vi "Main v0.95.vi"() -> ()   [LabVIEW 2017]
doc: "v0.85:\n- Counts for rejects and total\n\nv0.5:\n\n- Added Reject to Manual Mode\n- Send reject pallet cluster during manual mode\n- Run continuous manual happens only when no error has occured"
uses:
  Controls/Main Tabs v0.1.ctl
  Controls/Auto.ctl
  RT/Controls/Auto Delays.ctl
  RT/Controls/Auto Times.ctl
  Controls/UI Data.ctl
  support/Controls/Auto Stats.ctl
  support/Message Queue/Enqueue Message (Single).vi
  GV/Maintenance GV.vi
  <vilib>/Utility/error.llb/Error Cluster From Error Code.vi
  <vilib>/ErrorRing/Error Ring.xnode
  support/Message Queue/Message Queue.lvlib
  support/User Event - Stop/User Event - Stop.lvlib
panel:
  in  "Reject Pallets":T1
  out "Date-Time":string caption="Dip-Tube Assembly Automation (HMI) v0.9"
  out "Main Tab":T2
  in  "Autocycle":T3
  in  "Manual":bool
  in  "Parameters":bool
  in  "Maintenance":bool
  in  "BF Para":cluster{"Delay 1":u32, "Delay 2":u32}={"Delay 1"=1000, "Delay 2"=1000}
  in  "Reject Para":cluster{"Delay":u32}={"Delay"=400}
  in  "Meas. Para":T4={"Delay"=500.0, "Mean Length"=188.9, "Tolerance"=1.0}
  in  "PF Para":cluster{"Delay":u32, "Timeout":u32}={"Delay"=1000, "Timeout"=1000}
  in  "Tube Feeder Para":T5={"Delay"=400, "Delay 2"=250, "Max Attempts"=250}
  in  "Cutting Para":T6={"Delay"=400, "Delay 2"=250, "Delay 3"=250}
  in  "Agitator Para":cluster{"Delay":u32, "Timeout":u32}={"Delay"=400, "Timeout"=250}
  in  "Insertion Para":cluster{"Delay 1":u32, "Delay 2":u32}={"Delay 1"=1000, "Delay 2"=1000}
  in  "Save Para":bool
  in  "Home Para":bool
  out "OEE":dbl format="%#.1f"
  out "QUA":dbl=100.0 min=0.0 max=100.0 step=0.1
  in  "Ideal Time":dbl=2.0 min=0.0 max=100.0 step=0.1
  in  "AVL":dbl=100.0 min=0.0 max=100.0 step=0.1
  out "Rejects 2":u32
  in  "Reset MCount":bool
  in  "Enable BF?":bool
  in  "Enable Agitate?":bool
  in  "Enable Reject?":bool
  in  "Toggle Motor":bool
  in  "Continuous?":bool
  in  "Enable Measure?":bool
  in  "Enable Index?":bool
  in  "Enable PF?":bool
  in  "Auto Para":T7={"Agitator Delays"=[400, 250], "TF Delays"=[700, 800, 2], "Insertion Delays"=[100, 500], "Cutting Delays"=[300, 300, 100], "PF Delays"=[250, 30000], "Measur. Delays"=[500.0, 188.9, 1.0], "Reject Delays"=[500], "BF Delays"=[1000, 1000]}
  in  "Enable Cutting?":bool
  in  "Enable Insertion?":bool
  in  "Run Manual":bool
  in  "Enable TF?":bool
  in  "Home Manual":bool
  out "Status 2":T9
  out "Measurements":T10 {"Height 1" format="%#.2f"; "Height 2" format="%#.2f"; "Height 3" format="%#.2f"; "Height 4" format="%#.2f"}
  out "Output Count":u32 caption="Output\nCount"
  out "PRF":dbl=100.0 min=0.0 max=100.0 step=0.1
  out "Statuses":string[][](table)
  in  "All IO":bool
  in  "Stats":bool
  in  "Home AC":bool
  out "Status":string
  out "Count":u32 format="%06.0f"
  out "Cycle Time":dbl format="%0.2f"
  out "Rejects":u32 format="%06.0f"
  out "Output Chart":T11(graph)
  out "Reject Count":u32
  out "Total Count":u32
  out "Total Time":dbl caption="Total Effective Cycle Time (s)" format="%#.3f"
  out "Time Chart":T12(graph)
  out "OEE Chart":cluster{"1":dbl, "2":dbl, "3":dbl, "4":dbl}(graph)
  out "Measurement Chart":cluster{"1":dbl, "2":dbl, "3":dbl, "4":dbl}(graph)
  out "Timestamp":string caption="Date & Timestamp"
  out "Latest Measure.":T13 caption="Latest Measurements" {"Length 1 (mm)" format="%#.2f"}
  out "Auto Times":T8
  in  "Back Stats":bool
  out "OEE 2":T14 caption="Latest Measurements" {"AVL" format="%#.1f"; "PRF" format="%#.1f"; "QUA" format="%#.1f"; "OEE" format="%#.1f"}
  out "IAS 4":dbl format="%#.3f"
  out "IAS 3":dbl format="%#.3f"
  out "IAS 2":dbl format="%#.3f"
  out "IAS 1":dbl format="%#.3f"
  out "DI 1":T15
  out "DI 2":T16
  out "DO 1":T17
  in  "Back IO":bool
  in  "Exit":bool
  # "Vision Harmony Dip-Tube Assembly Automation"
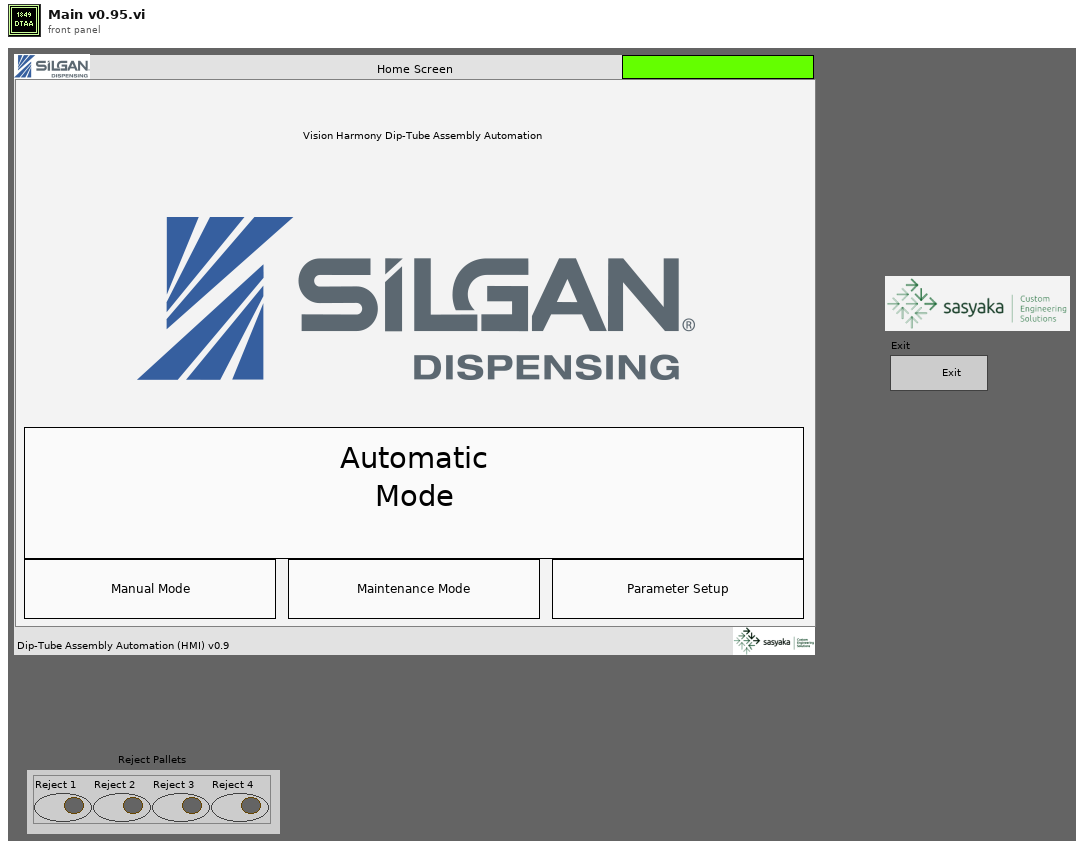
[diagram p1: front panel]
types:
  T1 = cluster{"Reject 1":bool, "Reject 2":bool, "Reject 3":bool, "Reject 4":bool}
  T2 = typedef "Main Tabs v0.1.ctl" = enum32{"Home Screen", "Parameter Setup", "Manual Mode", "Autocycle", "Autocycle Statistics", "Autocycle IOs"}
  T3 = typedef "Auto.ctl" = bool
  T4 = cluster{"Delay":dbl, "Mean Length":dbl, "Tolerance":dbl}
  T5 = cluster{"Delay":u32, "Delay 2":u32, "Max Attempts":u32}
  T6 = cluster{"Delay":u32, "Delay 2":u32, "Delay 3":u32}
  T7 = typedef "Auto Delays.ctl" = cluster{"Agitator Delays":u32[], "TF Delays":u32[], "Insertion Delays":u32[], "Cutting Delays":u32[], "PF Delays":u32[], "Measur. Delays":dbl[], "Reject Delays":u32[], "BF Delays":u32[]}
  T8 = typedef "Auto Times.ctl" = cluster{"Index Time":u32, "TF Time":u32, "Insertion Time":u32, "Cutting Time":u32, "PF Time":u32, "Meas. Time":u32, "Reject Time":u32}
  T9 = cluster{"Auto Times":T8, "error out":errorcluster}
  T10 = cluster{"Height 1":dbl, "Height 2":dbl, "Height 3":dbl, "Height 4":dbl}
  T11 = cluster{"OutputCount":u32, "Numeric Control":u32}
  T12 = cluster{"Index":dbl, "TF":dbl, "Insert":dbl, "Cutting":dbl, "PF":dbl, "Measure.":dbl, "Reject":dbl}
  T13 = cluster{"Length 1 (mm)":dbl, "Pallet 2 (mm)":dbl, "Pallet 3 (mm)":dbl, "Pallet 4 (mm)":dbl}
  T14 = cluster{"AVL":dbl, "PRF":dbl, "QUA":dbl, "OEE":dbl}
  T15 = cluster{"Machine_ON":bool, "E_stop ":bool, "SW_Pressure":bool, "SW_Start ":bool, "SW_Reset":bool, "SW_Stop":bool, "SW_Door":bool, "RS_Index_Rotary_CW":bool, "RS_Index_Rotary_CCW":bool, "RS_Index_Stopper _Rear":bool, "RS_Index_Output_Separator_Rear":bool, "PES_Index_Pallet_Sensor":bool, "PES_Index_Output_Part Sensor":bool, "ICS_BF_Low_Level_1":bool, "ICS_BF_Low_Level_2":bool, "ICS_BF_Pump_CNVR_Full_1":bool, "ICS_BF_Pump_CNVR_Full_2":bool, "ICS_BF_Pump_CNVR_Full_3":bool, "ICS_BF_Pump_CNVR_Full_4":bool, "PES_PC_Pump Presence_1":bool, "PES_PC_Pump Presence_2":bool, "PES_PC_Pump Presence_3":bool, "PES_PC_Pump Presence_4":bool, "RS_PC_Gating_Front":bool, "PES_Pump_Interference":bool, "PES_TF_Low_Level":bool, "PES_Tube Presence_1":bool, "PES_Tube Presence_2":bool, "PES_Tube Presence_3":bool, "PES_Tube Presence_4":bool, "DI1.30":bool, "DI1.31":bool}
  T16 = cluster{"RS_Agitatator_1_Rear ":bool, "RS_Agitatator_2_Rear ":bool, "RS_TF_Gating CYL_Rear":bool, "RS_Insertion_1_Rear":bool, "RS_Insertion_1_Front":bool, "RS_Insertion _2_Rear":bool, "RS_Insertion _2_Front":bool, "RS_Insertion _3_Rear":bool, "RS_Insertion _3_Front":bool, "RS_Insertion _4_Rear":bool, "RS_Insertion _4_Front":bool, "RS_Insertion_Clamp_Rear":bool, "RS_Cutting_Rear":bool, "RS_Cutting_Clamp _Rear":bool, "RS_Measurement_1_Rear":bool, "RS_Measurement_2_Rear":bool, "RS_Measurement_3_Rear":bool, "RS_Measurement_4_Rear":bool, "DI2.18":bool, "RS_Rejection_1_Rear":bool, "RS_Rejection_2_Rear":bool, "RS_Rejection_3_Rear":bool, "RS_Rejection_4_Rear":bool, "DI2.23":bool, "DI2.24":bool, "DI2.25":bool, "DI2.26":bool, "DI2.27":bool, "DI2.28":bool, "DI2.29":bool, "DI2.30":bool, "DI2.31":bool}
  T17 = cluster{"TL_Red":bool, "TL_Orange":bool, "TL_Green":bool, "TL_Buzzer":bool, "SOL_Index_Rotary_CW":bool, "SOL_Index_Rotary_CCW":bool, "SOL_Index_Stopper_Rear":bool, "SOL_OutputSeparator_Rear":bool, "Bowl  Feeder_ ON 1":bool, "Pump_CNVR_Motor _ON":bool, "SOL_PC_Gating_CYL_Rear":bool, "SOL_Tube_Feed_Agitatator":bool, "SOL_Tube_Feed_Gating_CYL":bool, "SOL_Insertion _CYL":bool, "SOL_Insertion_Clamp_CYL":bool, "SOL_Cutting_CYL":bool, "SOL_Cutting_Clamp_CYL":bool, "SOL_Insertion_Air_Nozzle":bool, "SOL_Measurement_CYL":bool, "DO1.19":bool, "SOL_Rejection CYL_1":bool, "SOL_Rejection CYL_2":bool, "SOL_Rejection CYL_3":bool, "SOL_Rejection CYL_4":bool, "Bowl  Feeder_ ON 2":bool, "SOL_BF_BlowerON":bool, "SOL_BF1_Track1":bool, "SOL_BF1_Track2":bool, "SOL_BF2_Track1":bool, "SOL_BF2_Track2":bool, "DO1.30":bool, "DO1.31":bool}
  T18 = typedef "UI Data.ctl" = cluster{"Main Tab":refnum<vi>}
  T19 = typedef "Message Queue.lvlib/All Message Queues.ctl" = cluster{"UI":refnum<queue>}
  T20 = enum8{"Enabled", "Disabled", "Disabled and Grayed Out"}
  T21 = cluster{"Array":string[][], "Machine Status":string}
  T22 = typedef "Auto Stats.ctl" = cluster{"Time":timestamp, "OEE":cluster{"AVL":dbl, "PRF":dbl, "QUA":dbl, "OEE":dbl}, "Auto Times":T8, "Counts out":cluster{"OutputCount":u32, "RejectCount":u32}, "Measurements":cluster{"1":dbl, "2":dbl, "3":dbl, "4":dbl}, "Outputs":cluster{"OutputCount":u32, "Numeric Control":u32}}
  T23 = cluster{"Auto Times":T8, "Results":cluster{"Measurements":cluster{"1":dbl, "2":dbl, "3":dbl, "4":dbl}, "Reject Pallets":cluster{"Reject 1":bool, "Reject 2":bool, "Reject 3":bool, "Reject 4":bool}}, "OutputCount":u32, "error out":errorcluster}
  T24 = cluster{"Agitator Delays[0]":u32, "Agitator Delays[1]":u32}
  T25 = cluster{"TF Delays[0]":u32, "TF Delays[1]":u32, "TF Delays[2]":u32}
  T26 = cluster{"Insertion Delays[0]":u32, "Insertion Delays[1]":u32}
  T27 = cluster{"Cutting Delays[0]":u32, "Cutting Delays[1]":u32, "Cutting Delays[2]":u32}
  T28 = cluster{"Measur. Delays[0]":dbl, "Measur. Delays[1]":dbl, "Measur. Delays[2]":dbl}
  T29 = typedef "All Inputs.ctl" = cluster{"DI 1":cluster{"Machine_ON":bool, "E_stop ":bool, "SW_Pressure":bool, "SW_Start ":bool, "SW_Reset":bool, "SW_Stop":bool, "SW_Door":bool, "RS_Index_Rotary_CW":bool, "RS_Index_Rotary_CCW":bool, "RS_Index_Stopper _Rear":bool, "RS_Index_Output_Separator_Rear":bool, "PES_Index_Pallet_Sensor":bool, "PES_Index_Output_Part Sensor":bool, "ICS_BF_Low_Level_1":bool, "ICS_BF_Low_Level_2":bool, "ICS_BF_Pump_CNVR_Full_1":bool, "ICS_BF_Pump_CNVR_Full_2":bool, "ICS_BF_Pump_CNVR_Full_3":bool, "ICS_BF_Pump_CNVR_Full_4":bool, "PES_PC_Pump Presence_1":bool, "PES_PC_Pump Presence_2":bool, "PES_PC_Pump Presence_3":bool, "PES_PC_Pump Presence_4":bool, "RS_PC_Gating_Front":bool, "PES_Pump_Interference":bool, "PES_TF_Low_Level":bool, "PES_Tube Presence_1":bool, "PES_Tube Presence_2":bool, "PES_Tube Presence_3":bool, "PES_Tube Presence_4":bool, "DI1.30":bool, "DI1.31":bool}, "DI 2":cluster{"RS_Agitatator_1_Rear ":bool, "RS_Agitatator_2_Rear ":bool, "RS_TF_Gating CYL_Rear":bool, "RS_Insertion_1_Rear":bool, "RS_Insertion_1_Front":bool, "RS_Insertion _2_Rear":bool, "RS_Insertion _2_Front":bool, "RS_Insertion _3_Rear":bool, "RS_Insertion _3_Front":bool, "RS_Insertion _4_Rear":bool, "RS_Insertion _4_Front":bool, "RS_Insertion_Clamp_Rear":bool, "RS_Cutting_Rear":bool, "RS_Cutting_Clamp _Rear":bool, "RS_Measurement_1_Rear":bool, "RS_Measurement_2_Rear":bool, "RS_Measurement_3_Rear":bool, "RS_Measurement_4_Rear":bool, "RS_Measure_Clamp_Rear":bool, "RS_Rejection_1_Rear":bool, "RS_Rejection_2_Rear":bool, "RS_Rejection_3_Rear":bool, "RS_Rejection_4_Rear":bool, "DI2.23":bool, "DI2.24":bool, "DI2.25":bool, "DI2.26":bool, "DI2.27":bool, "DI2.28":bool, "DI2.29":bool, "DI2.30":bool, "DI2.31":bool}, "IAS 1":dbl, "IAS 2":dbl, "IAS 3":dbl, "IAS 4":dbl, "DO 1":cluster{"TL_Red":bool, "TL_Orange":bool, "TL_Green":bool, "TL_Buzzer":bool, "SOL_Index_Rotary_CW":bool, "SOL_Index_CNVR_Rotary_CCW":bool, "SOL_Index_CNVR_Stopper_Rear":bool, "SOL_Index_CNVR_Output _Separator _Rear":bool, "Bowl  Feeder_ ON 1":bool, "Pump_CNVR_Motor _ON":bool, "SOL_PC_Gating_CYL_Rear":bool, "SOL_Tube_Feed_Agitatator":bool, "SOL_Tube_Feed_Gating_CYL":bool, "SOL_Insertion _CYL":bool, "SOL_Insertion_Clamp_CYL":bool, "SOL_Cutting_CYL":bool, "SOL_Cutting_Clamp_CYL":bool, "SOL_Insertion_Air_Nozzle":bool, "SOL_Measurement_CYL":bool, "DO1.19":bool, "SOL_Rejection CYL_1":bool, "SOL_Rejection CYL_2":bool, "SOL_Rejection CYL_3":bool, "SOL_Rejection CYL_4":bool, "Bowl  Feeder_ ON 2":bool, "SOL_BF_BlowerON":bool, "SOL_BF1_Track1":bool, "SOL_BF1_Track2":bool, "SOL_BF2_Track1":bool, "SOL_BF2_Track2":bool, "DO1.30":bool, "DO1.31":bool}}
  T30 = cluster{"RS_Agitatator_1_Rear ":bool, "RS_Agitatator_2_Rear ":bool, "RS_TF_Gating CYL_Rear":bool, "RS_Insertion_1_Rear":bool, "RS_Insertion_1_Front":bool, "RS_Insertion _2_Rear":bool, "RS_Insertion _2_Front":bool, "RS_Insertion _3_Rear":bool, "RS_Insertion _3_Front":bool, "RS_Insertion _4_Rear":bool, "RS_Insertion _4_Front":bool, "RS_Insertion_Clamp_Rear":bool, "RS_Cutting_Rear":bool, "RS_Cutting_Clamp _Rear":bool, "RS_Measurement_1_Rear":bool, "RS_Measurement_2_Rear":bool, "RS_Measurement_3_Rear":bool, "RS_Measurement_4_Rear":bool, "RS_Measure_Clamp_Rear":bool, "RS_Rejection_1_Rear":bool, "RS_Rejection_2_Rear":bool, "RS_Rejection_3_Rear":bool, "RS_Rejection_4_Rear":bool, "DI2.23":bool, "DI2.24":bool, "DI2.25":bool, "DI2.26":bool, "DI2.27":bool, "DI2.28":bool, "DI2.29":bool, "DI2.30":bool, "DI2.31":bool}
  T31 = cluster{"TL_Red":bool, "TL_Orange":bool, "TL_Green":bool, "TL_Buzzer":bool, "SOL_Index_Rotary_CW":bool, "SOL_Index_CNVR_Rotary_CCW":bool, "SOL_Index_CNVR_Stopper_Rear":bool, "SOL_Index_CNVR_Output _Separator _Rear":bool, "Bowl  Feeder_ ON 1":bool, "Pump_CNVR_Motor _ON":bool, "SOL_PC_Gating_CYL_Rear":bool, "SOL_Tube_Feed_Agitatator":bool, "SOL_Tube_Feed_Gating_CYL":bool, "SOL_Insertion _CYL":bool, "SOL_Insertion_Clamp_CYL":bool, "SOL_Cutting_CYL":bool, "SOL_Cutting_Clamp_CYL":bool, "SOL_Insertion_Air_Nozzle":bool, "SOL_Measurement_CYL":bool, "DO1.19":bool, "SOL_Rejection CYL_1":bool, "SOL_Rejection CYL_2":bool, "SOL_Rejection CYL_3":bool, "SOL_Rejection CYL_4":bool, "Bowl  Feeder_ ON 2":bool, "SOL_BF_BlowerON":bool, "SOL_BF1_Track1":bool, "SOL_BF1_Track2":bool, "SOL_BF2_Track1":bool, "SOL_BF2_Track2":bool, "DO1.30":bool, "DO1.31":bool}
  T32 = cluster{"Auto Para":T7, "Reject Pallets":cluster{"Reject 1":bool, "Reject 2":bool, "Reject 3":bool, "Reject 4":bool}}
  T33 = cluster{"Measurements":cluster{"1":dbl, "2":dbl, "3":dbl, "4":dbl}, "Reject Pallets":cluster{"Reject 1":bool, "Reject 2":bool, "Reject 3":bool, "Reject 4":bool}}
  T34 = cluster{"Reject Pallets":cluster{"Reject 1":bool, "Reject 2":bool, "Reject 3":bool, "Reject 4":bool}, "Measurements":cluster{"1":dbl, "2":dbl, "3":dbl, "4":dbl}}
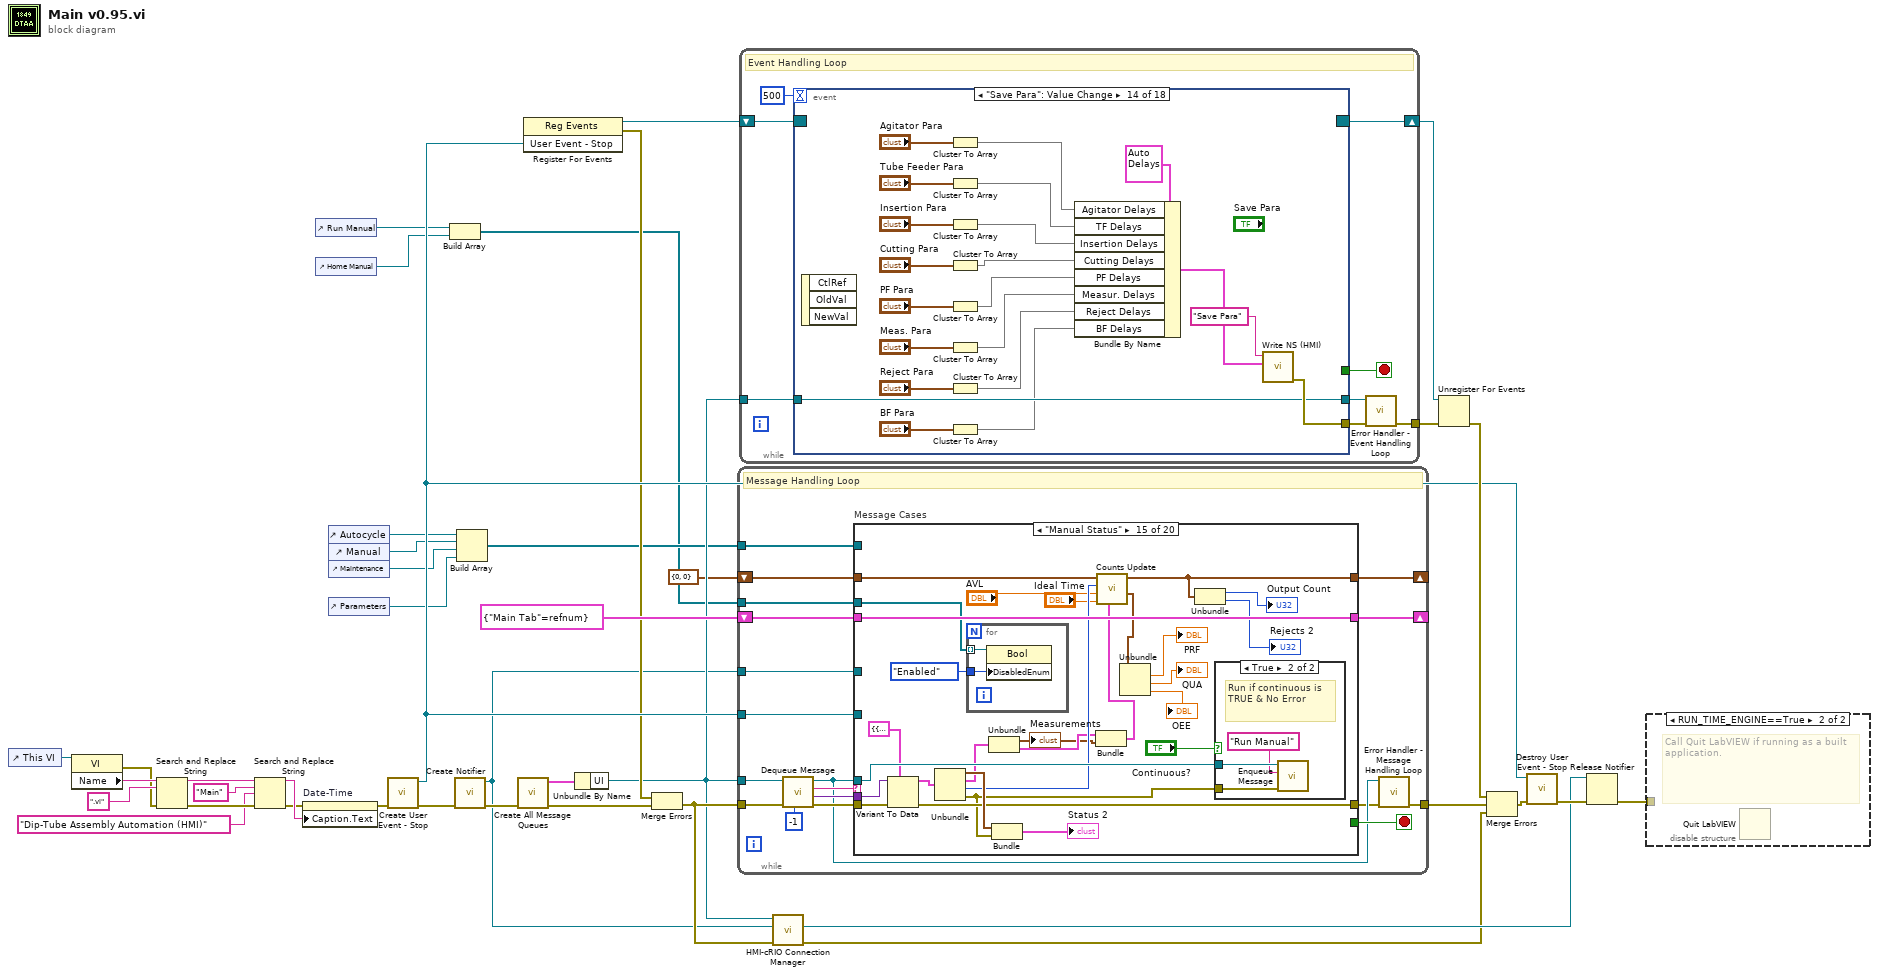
[diagram p0: block diagram]
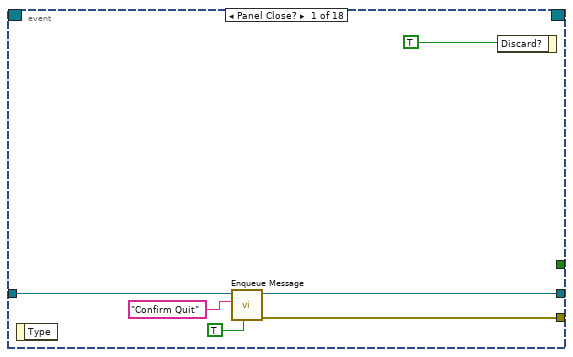
[diagram p2: hidden frame]
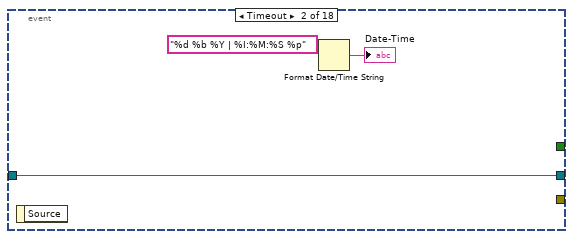
[diagram p3: hidden frame]
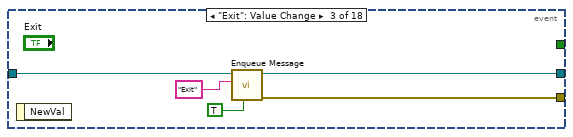
[diagram p4: hidden frame]
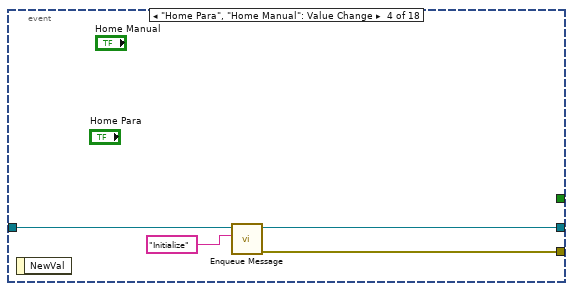
[diagram p5: hidden frame]
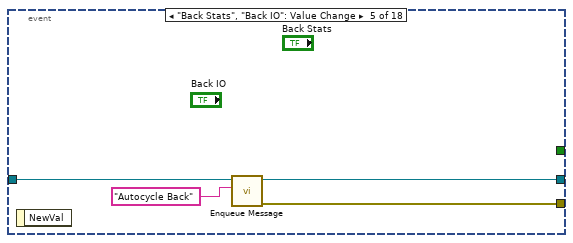
[diagram p6: hidden frame]
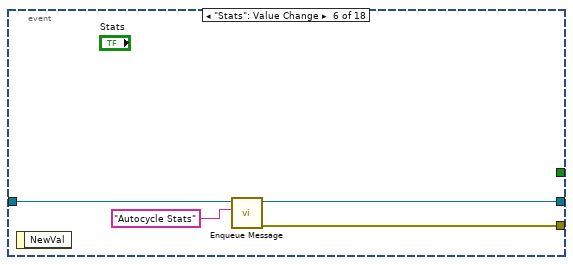
[diagram p7: hidden frame]
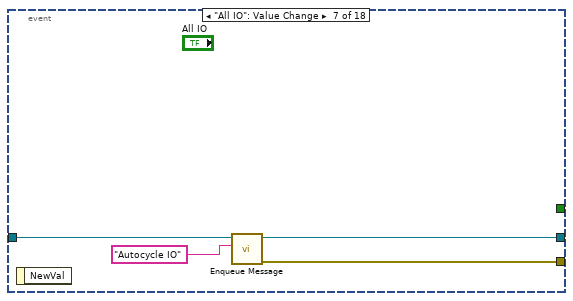
[diagram p8: hidden frame]
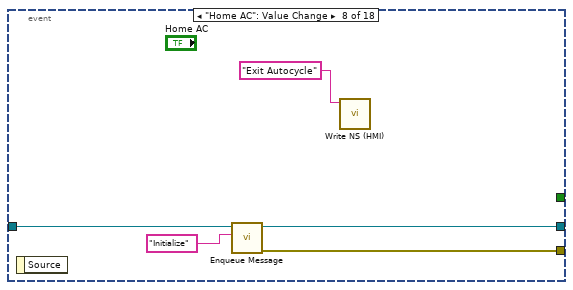
[diagram p9: hidden frame]
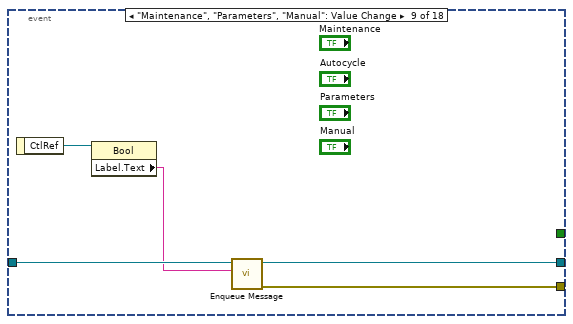
[diagram p10: hidden frame]
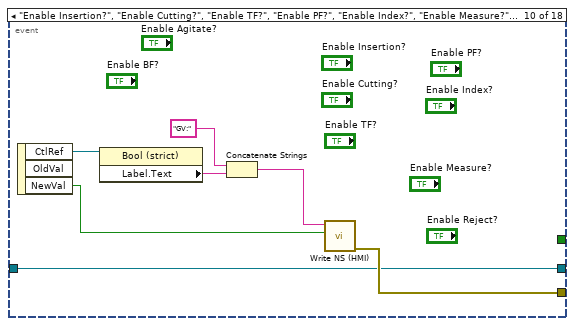
[diagram p11: hidden frame]
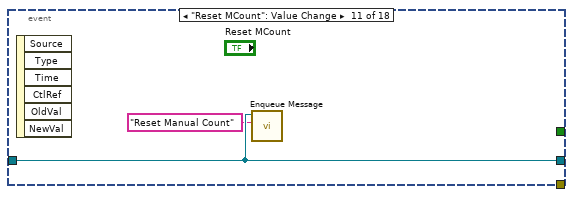
[diagram p12: hidden frame]
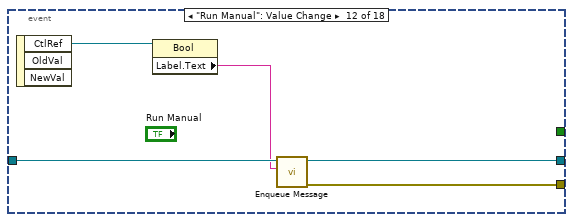
[diagram p13: hidden frame]
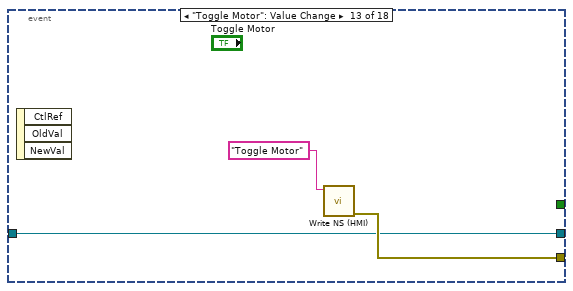
[diagram p14: hidden frame]
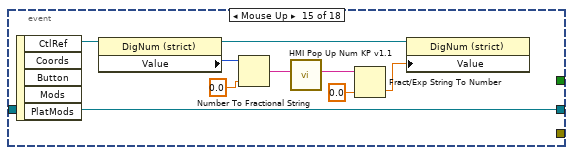
[diagram p15: hidden frame]
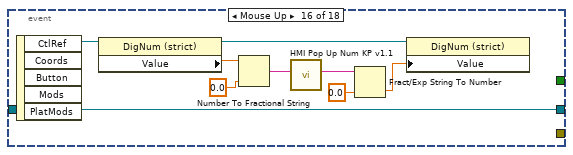
[diagram p16: hidden frame]
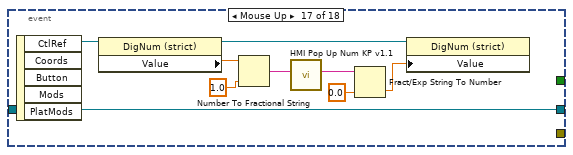
[diagram p17: hidden frame]
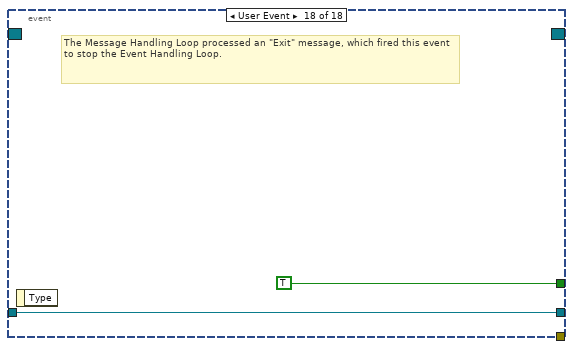
[diagram p18: hidden frame]
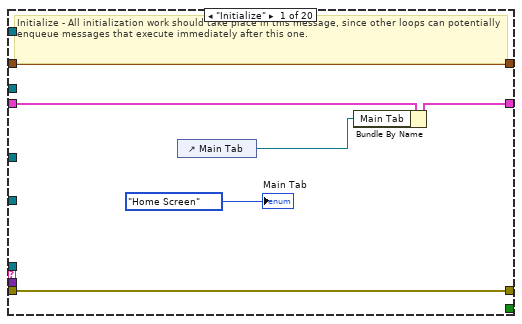
[diagram p19: hidden frame]
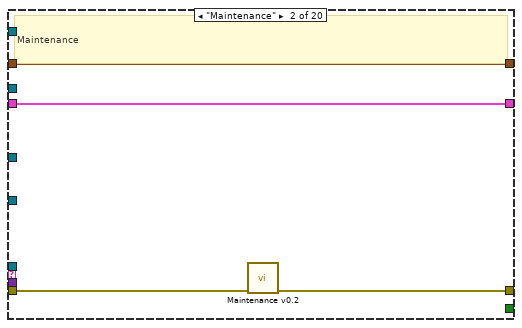
[diagram p20: hidden frame]
diagram:
  n1 = control-ref of="This VI"() -> (w9:refnum<vi>)
  n2 = property class="VI"(reference=w9) -> (error out=w8:errorcluster, "Name"=w15:string)  [unwired: 1 in, 1 out]
  n3 = Search and Replace String(input string=w15, search string=".vi", error in=w8) -> (result string=w13:string, error out=w12:errorcluster)  [unwired: 5 in, 2 out]
  n4 = Search and Replace String(input string=w13, search string="Main", replace string="Dip-Tube Assembly Automation (HMI)" ("replace string (\"\")"), error in=w12) -> (result string=w7:string, error out=w6:errorcluster)  [unwired: 4 in, 2 out]
  n5 = property on="Date-Time" class="Str"(error in=w6, "Caption.Text"=w7) -> (error out=w5:errorcluster)  [unwired: 1 in, 1 out]
  n6 = control-ref of="Run Manual"() -> (w4:refnum<vi>)
  n7 = control-ref of="Home Manual"() -> (w3:refnum<vi>)
  n8 = control-ref of="Autocycle"() -> (w20:refnum<vi>)
  n9 = control-ref of="Manual"() -> (w19:refnum<vi>)
  n10 = control-ref of="Maintenance"() -> (w18:refnum<vi>)
  n11 = control-ref of="Parameters"() -> (w17:refnum<vi>)
  n12 = call "Create User Event - Stop.vi"("error in (no error)"=w5) -> ("error out"=w27:errorcluster, "User Event - Stop"=w31:refnum<user-event>)  [unwired: 9 in]
  n13 = Build Array(w4, w3) -> (w2:refnum<vi>[])
  n14 = call "Create Notifier.vi"("error in (no error)"=w27) -> ("error out"=w26:errorcluster, "notifier out"=w21:refnum<notifier>)  [unwired: 9 in]
  n15 = Build Array(w20, w19, w18, w17) -> (w16:refnum<vi>[])
  n16 = call "Create All Message Queues.vi"("error in (no error)"=w26) -> ("error out"=w40:errorcluster, "Message Queues out"=w39:T19)  [unwired: 9 in]
  n17 = register-events(w31) -> (reference out=w32:refnum<event-registration>, error out=w30:errorcluster)  [unwired: 2 in]
  n18 = Unbundle By Name(w39) -> ("UI"=w28:refnum<queue>)
  n19 = Merge Errors(w30, w40) -> (w29:errorcluster)
  n20 = while {
    tunnel: w28 -> [w51]
    shift-right: [w58] -> _
    shift-left: T18 {"Main Tab"=refnum} ("Data Cluster") -> [w41]
    tunnel: w31 -> [w56]
    tunnel: w29 -> [w55]
    tunnel: [w49] -> w38
    tunnel: w21 -> [w46]
    tunnel: w16 -> [w45]
    tunnel: w2 -> [w44]
    shift-right: [w42] -> _
    shift-left: cluster{"OutputCount":u32, "RejectCount":u32} {"OutputCount"=0, "RejectCount"=0} -> [w43]
    stop <- w57 stop-if-true
    # "Message Handling Loop"
    n21 = call "Dequeue Message.vi"("timeout"=-1, "error in (no error)"=w55, "Message Queue"=w51) -> ("error out"=w54:errorcluster, "Message Data"=w52:variant, "Message"=w53:string, "dup Message Queue"=w50:refnum<queue>)  [unwired: 5 in]
    n22 = case "Message Cases" shown="\"Manual Status\"" w53 {
      selector: w53 -> [_ _ _ _ _ _ _ _ _ _ _ _ _ _ _ _ _ _ _ w296]
      tunnel: w50 -> [_ _ _ _ _ _ _ _ _ w154 w162 _ _ _ w245 _ _ w275 w294 _]
      tunnel: w54 -> [w64 w67 w80 w86 w112 w127 w134 w144 w149 w156 w170 w192 w211 w221 w253 w263 w271 w279 w287 _]
      tunnel: [w64 w66 w79 w85 w111 w127 w133 w144 w149 w155 w169 w193 w212 w223 w244 w263 w265 w277 w290 w297] -> w48
      tunnel: w41 -> [w63 w68 w82 w91 w114 w126 w130 w148 w153 w161 w167 w194 w213 w224 w254 w262 w270 w278 w293 w298]
      tunnel: [w62 w68 w82 w91 w114 w126 w130 w148 w153 w161 w167 w194 w213 w224 w254 w262 w270 w278 w293 w298] -> w58
      tunnel: [_ _ _ _ _ _ _ _ _ _ _ _ _ _ _ _ _ _ TRUE _] -> w57
      tunnel: w52 -> [_ _ w78 _ w110 _ _ _ _ _ _ w191 w210 _ w252 _ w269 _ w284 _]
      tunnel: w56 -> [_ _ _ _ _ _ _ _ _ _ _ _ _ _ _ _ _ _ w289 _]
      tunnel: w46 -> [_ _ _ _ _ _ _ _ _ _ _ _ _ _ _ _ _ _ w283 _]
      tunnel: w45 -> [_ _ w74 _ _ _ _ _ _ _ _ _ _ _ _ _ _ _ _ _]
      tunnel: w44 -> [_ _ _ _ _ _ _ _ _ _ _ _ _ w218 w250 _ _ _ _ _]
      tunnel: w43 -> [w59 w65 w69 w88 w113 w115 w135 w145 w150 w158 w171 w189 w208 w214 w243 _ w264 w272 w280 w295]
      tunnel: [w59 w65 w69 w88 w113 w115 w135 w145 w150 w158 w171 w189 w208 w214 w238 cluster{"OutputCount":u32, "RejectCount":u32} {"OutputCount"=0, "RejectCount"=0} w264 w272 w280 w295] -> w42
      frame "Initialize" {
        # "Initialize - All initialization work should take place in this message, since other loops can potentially enqueue messages that execute immediately after this one."
        n23 = control-ref of="Main Tab"() -> (w61:refnum<vi>)
        n24 = Bundle By Name(cluster=w63, "Main Tab"=w61) -> (w62:T18)
        "Main Tab" <- Main_Tabs_v0.1."Home Screen" ("Main Tab")
      }
      frame "Maintenance" {
        # "Maintenance"
        n25 = call "Maintenance v0.2.vi"("Error In"=w67) -> ("Error out"=w66:errorcluster)  [unwired: 10 in]
      }
      frame "Connection" {
        n26 = Variant To Data(error in=w80, type=FALSE, Variant=w78) -> (data=w73:bool, error out=w79:errorcluster)
        n27 = Select(t=u32 6618880 ("Text.Text Colors:BG Color"), s=w73, f=u32 16762112 ("Text.Text Colors:BG Color")) -> (s? t:f=w75:u32)
        n28 = property on="Date-Time" class="Str"("Text.BGColor"=w75) -> ()  [unwired: 2 in, 2 out]
        n29 = Select(t=T20."Enabled" ("Disabled"), s=w73, f=T20."Disabled and Grayed Out") -> (s? t:f=w71:T20)
        n30 = for {
          tunnel: w74 -> [w84] mode=indexing
          tunnel: w71 -> [w83]
          n31 = property class="Bool"(reference=w84, "DisabledEnum"=w83) -> ()  [unwired: 1 in, 2 out]
        }
      }
      frame "Parameters" {
        # "Parameters"
        n32 = Unbundle By Name(w91) -> ("Main Tab"=w90:refnum<vi>)
        n33 = call "Write NS (HMI).vi"("error in (no error)"=w86, "Message"="Enter Para") -> ("error out"=w85:errorcluster)  [unwired: 9 in]
        n34 = property class="TabCtl"(reference=w90, "Value"=Main_Tabs_v0.1."Parameter Setup" ("Main Tab")) -> ()  [unwired: 1 in, 2 out]
      }
      frame "Current Para" {
        # "Parameters"
        n35 = Variant To Data(error in=w112, type=T7 {"Agitator Delays"=[1000], "TF Delays"=[1000], "Insertion Delays"=[1000], "Cutting Delays"=[1000], "PF Delays"=[1000], "Measur. Delays"=[1000.0], "Reject Delays"=[1000], "BF Delays"=[1000]} ("Auto Para"), Variant=w110) -> (data=w108:T7, error out=w111:errorcluster)
        n36 = Unbundle(w108) -> ("Agitator Delays"=w107:u32[], "TF Delays"=w106:u32[], "Insertion Delays"=w105:u32[], "Cutting Delays"=w104:u32[], "PF Delays"=w103:u32[], "Measur. Delays"=w102:dbl[], "Reject Delays"=w101:u32[], "BF Delays"=w100:u32[])
        n37 = property on="Auto Para" class="Clust (strict)"("Value"=w108) -> ()  [unwired: 2 in, 2 out]
        n38 = Array To Cluster(array=w107) -> (cluster=w99:T24)
        n39 = Array To Cluster(array=w106) -> (cluster=w98:T25)
        n40 = Array To Cluster(array=w105) -> (cluster=w97:T26)
        n41 = Array To Cluster(array=w104) -> (cluster=w96:T27)
        n42 = Array To Cluster(array=w103) -> (cluster=w95:cluster{"PF Delays[0]":u32, "PF Delays[1]":u32})
        n43 = Array To Cluster(array=w102) -> (cluster=w94:T28)
        n44 = Array To Cluster(array=w101) -> (cluster=w93:cluster{"Reject Delays[0]":u32})
        n45 = Array To Cluster(array=w100) -> (cluster=w92:cluster{"BF Delays[0]":u32, "BF Delays[1]":u32})
        n46 = property on="Agitator Para" class="Clust (strict)"("Value"=w99) -> ()  [unwired: 2 in, 2 out]
        n47 = property on="Tube Feeder Para" class="Clust (strict)"("Value"=w98) -> ()  [unwired: 2 in, 2 out]
        n48 = property on="Insertion Para" class="Clust (strict)"("Value"=w97) -> ()  [unwired: 2 in, 2 out]
        n49 = property on="Cutting Para" class="Clust (strict)"("Value"=w96) -> ()  [unwired: 2 in, 2 out]
        n50 = property on="PF Para" class="Clust (strict)"("Value"=w95) -> ()  [unwired: 2 in, 2 out]
        n51 = property on="Meas. Para" class="Clust (strict)"("Value"=w94) -> ()  [unwired: 2 in, 2 out]
        n52 = property on="Reject Para" class="Clust (strict)"("Value"=w93) -> ()  [unwired: 2 in, 2 out]
        n53 = property on="BF Para" class="Clust (strict)"("Value"=w92) -> ()  [unwired: 2 in, 2 out]
      }
      frame "Manual" {
        # "Parameters"
        n54 = control-ref of="Enable Index?"() -> (w123:refnum<vi>)
        n55 = control-ref of="Enable PF?"() -> (w122:refnum<vi>)
        n56 = control-ref of="Enable Cutting?"() -> (w121:refnum<vi>)
        n57 = control-ref of="Enable Insertion?"() -> (w120:refnum<vi>)
        n58 = control-ref of="Enable TF?"() -> (w119:refnum<vi>)
        n59 = control-ref of="Enable Measure?"() -> (w117:refnum<vi>)
        n60 = control-ref of="Enable Reject?"() -> (w116:refnum<vi>)
        n61 = Build Array(w123, w122, w121, w120, w119, w117, w116) -> (w118:refnum<vi>[])
        n62 = for {
          tunnel: w118 -> [w129] mode=indexing
          n63 = property class="Bool (strict)"(reference=w129, "Val(Sgnl)"=FALSE ("Value (Signaling)")) -> ()  [unwired: 1 in, 2 out]
        }
        n64 = Unbundle By Name(w126) -> ("Main Tab"=w125:refnum<vi>)
        n65 = property class="TabCtl"(reference=w125, "Value"=Main_Tabs_v0.1."Manual Mode" ("Main Tab")) -> ()  [unwired: 1 in, 2 out]
      }
      frame "Autocycle" {
        # "Parameters"
        n66 = call "Select Model.vi"() -> ("Cancel out"=w131:bool, "Model out"=w132:string)  [unwired: 10 in]
        n67 = case shown="False" w131 {
          tunnel: w134 -> [w141 w143]
          tunnel: [w140 w143] -> w133
          tunnel: w132 -> [w139 _]
          tunnel: w130 -> [w136 _]
          frame False {
            n68 = Unbundle By Name(w136) -> ("Main Tab"=w138:refnum<vi>)
            n69 = call "Write NS (HMI).vi"("error in (no error)"=w141, "Message Data"=w139, "Message"="Autocycle") -> ("error out"=w140:errorcluster)  [unwired: 8 in]
            n70 = property class="TabCtl"(reference=w138, "Value"=Main_Tabs_v0.1."Autocycle" ("Main Tab")) -> ()  [unwired: 1 in, 2 out]
          }
          frame True {
          }
        }
      }
      frame "Autocycle Back" {
        # "Parameters"
        n71 = Unbundle By Name(w148) -> ("Main Tab"=w147:refnum<vi>)
        n72 = property class="TabCtl"(reference=w147, "Value"=Main_Tabs_v0.1."Autocycle" ("Main Tab")) -> ()  [unwired: 1 in, 2 out]
      }
      frame "Autocycle Stats" {
        # "Parameters"
        n73 = Unbundle By Name(w153) -> ("Main Tab"=w152:refnum<vi>)
        n74 = property class="TabCtl"(reference=w152, "Value"=Main_Tabs_v0.1."Autocycle Statistics" ("Main Tab")) -> ()  [unwired: 1 in, 2 out]
      }
      frame "Autocycle IO" {
        # "Parameters"
        n75 = Unbundle By Name(w161) -> ("Main Tab"=w160:refnum<vi>)
        n76 = property class="TabCtl"(reference=w160, "Value"=Main_Tabs_v0.1."Autocycle IOs" ("Main Tab")) -> ()  [unwired: 1 in, 2 out]
        n77 = call-poly "Enqueue Message.vi"("error in (no error)"=w156, "Message"="Update IO", "Message Queue"=w154) -> ("error out"=w155:errorcluster)  [unwired: 7 in, 1 out]
      }
      frame "Update IO" {
        n78 = Unbundle By Name(w167) -> ("Main Tab"=w168:refnum<vi>)
        n79 = Wait (ms)(milliseconds to wait=u32 200) -> ()  [unwired: 1 out]
        n80 = property class="TabCtl"(reference=w168) -> ("Value"=w166:variant)  [unwired: 1 in, 2 out]
        n81 = Variant To Data(type=Main_Tabs_v0.1."Autocycle IOs" ("Main Tab"), Variant=w166) -> (data=w163:T2)  [unwired: 1 in, 1 out]
        n82 = global read "Maintenance GV.vi" "All IO"() -> (w172:T29)
        n83 = case shown="\"Autocycle IOs\"" w163 {
          tunnel: w170 -> [w180 w183]
          tunnel: [w180 w182] -> w169
          tunnel: w162 -> [_ w181]
          frame Default {
          }
          frame "Autocycle IOs" {
            n84 = call-poly "Enqueue Message.vi"("error in (no error)"=w183, "Message"="Update IO", "Message Queue"=w181) -> ("error out"=w182:errorcluster)  [unwired: 7 in, 1 out]
          }
        }
        n85 = Unbundle(w172) -> ("DI 1"=→"DI 1":T15, "DI 2"=→"DI 2":T30, "IAS 1"=→"IAS 1":dbl, "IAS 2"=→"IAS 2":dbl, "IAS 3"=→"IAS 3":dbl, "IAS 4"=→"IAS 4":dbl, "DO 1"=→"DO 1":T31)
      }
      frame "Update UI" {
        # "Update Display - Convert the message data to a string to display in the Data Display indicator."
        n86 = Variant To Data(error in=w192, type=T21 {"Array"=[], "Machine Status"=""} ("Status Cluster"), Variant=w191) -> (data=w187:T21, error out=w190:errorcluster)
        n87 = Unbundle(w187) -> ("Array"=→"Statuses":string[][], "Machine Status"=→"Status":string)
        n88 = Merge Errors(w190) -> (w193:errorcluster)
      }
      frame "Autocycle Log" {
        # "Update Display - Convert the message data to a string to display in the Data Display indicator."
        n89 = Variant To Data(error in=w211, type=T22 {"Time"=timestamp(0 s since 1904-01-01), "OEE"={"AVL"=100.0, "PRF"=100.0, "QUA"=100.0, "OEE"=0.0}, "Auto Times"={"Index Time"=0, "TF Time"=0, "Insertion Time"=0, "Cutting Time"=0, "PF Time"=0, "Meas. Time"=0, "Reject Time"=0}, "Counts out"={"OutputCount"=0, "RejectCount"=0}, "Measurements"={"1"=0.0, "2"=0.0, "3"=0.0, "4"=0.0}, "Outputs"={"OutputCount"=0, "Numeric Control"=0}} ("Auto Stats"), Variant=w210) -> (data=w206:T22, error out=w209:errorcluster)
        n90 = call "Stats Unbundle.vi"("Auto Stats"=w206) -> ("Cycle Time"=→"Cycle Time" →"Total Time":dbl, "RejectCount"=→"Rejects" →"Reject Count":u32, "OutputCount"=→"Count" →"Total Count":u32, "Total Times"=→"Time Chart":T12)  [unwired: 7 in]
        n91 = Unbundle(w206) -> ("Time"=w204:timestamp, "OEE"=→"OEE Chart" →"OEE 2":T14, "Auto Times"=→"Auto Times":T8, "Measurements"=→"Latest Measure." →"Measurement Chart":cluster{"1":dbl, "2":dbl, "3":dbl, "4":dbl}, "Outputs"=→"Output Chart":T11)  [unwired: 1 out]
        n92 = Format Date/Time String(time format string (%c)="%d-%m-%Y | %H:%M:%S%3u", seconds (now)=w204) -> (date/time string=→"Timestamp":string)  [unwired: 1 in]
        n93 = Merge Errors(w209) -> (w212:errorcluster)
      }
      frame "Run Manual" {
        # "Update Manual mode"
        n94 = Bundle("Auto Para"="Auto Para", "Reject Pallets"="Reject Pallets") -> (w215:T32)  [unwired: 1 in]
        n95 = for {
          tunnel: w218 -> [w226] mode=indexing
          tunnel: T20."Disabled and Grayed Out" ("Disabled") -> [w225]
          n96 = property class="Bool"(reference=w226, "DisabledEnum"=w225) -> ()  [unwired: 1 in, 2 out]
        }
        n97 = call "Write NS (HMI).vi"("error in (no error)"=w221, "Message Data"=w215, "Message"="Manual Run") -> ("error out"=w220:errorcluster)  [unwired: 8 in]
        n98 = Merge Errors(w220) -> (w223:errorcluster)
      }
      frame "Manual Status" {
        n99 = Variant To Data(error in=w253, type=T23 {"Auto Times"={"Index Time"=0, "TF Time"=0, "Insertion Time"=0, "Cutting Time"=0, "PF Time"=0, "Meas. Time"=0, "Reject Time"=0}, "Results"={"Measurements"={"1"=0.0, "2"=0.0, "3"=0.0, "4"=0.0}, "Reject Pallets"={"Reject 1"=FALSE, "Reject 2"=FALSE, "Reject 3"=FALSE, "Reject 4"=FALSE}}, "OutputCount"=0, "error out"={"status"=FALSE, "code"=0, "source"=""}} ("cluster"), Variant=w252) -> (data=w249:T23, error out=w244:errorcluster)
        n100 = Unbundle(w249) -> ("Auto Times"=w248:T8, "Results"=w240:T33, "OutputCount"=w239:u32, "error out"=w242:errorcluster)
        n101 = for {
          tunnel: w250 -> [w259] mode=indexing
          tunnel: T20."Enabled" ("Disabled") -> [w258]
          n102 = property class="Bool"(reference=w259, "DisabledEnum"=w258) -> ()  [unwired: 1 in, 2 out]
        }
        n103 = Unbundle(w240) -> ("Measurements"=w228:cluster{"1":dbl, "2":dbl, "3":dbl, "4":dbl}, "Reject Pallets"=w229:T1)
        "Measurements" <- w228
        n104 = Bundle("Auto Times"=w248, "error out"=w242) -> (→"Status 2":T9)  [unwired: 1 in]
        n105 = Bundle("Reject Pallets"=w229, "Measurements"=w228) -> (w227:T34)  [unwired: 1 in]
        n106 = call "Counts Update.vi"("output cluster"=w227, "Desired Cycle Time (s)"="Ideal Time", "AVL"="AVL", "OutputCount"=w239, "Counts in"=w243) -> ("OEE"=w233:T14, "Counts out"=w238:cluster{"OutputCount":u32, "RejectCount":u32})  [unwired: 4 in, 1 out]
        n107 = Unbundle(w233) -> ("PRF"=→"PRF":dbl, "QUA"=→"QUA":dbl, "OEE"=→"OEE":dbl)  [unwired: 1 out]
        n108 = Unbundle(w238) -> ("OutputCount"=→"Output Count":u32, "RejectCount"=→"Rejects 2":u32)
        n109 = case shown="True" "Continuous?" {
          tunnel: w245 -> [_ w257]
          tunnel: w242 -> [_ w256]
          frame False {
          }
          frame True {
            # "Run if continuous is TRUE & No Error"
            n110 = call-poly "Enqueue Message.vi"("error in (no error)"=w256, "Message"="Run Manual", "Message Queue"=w257) -> ()  [unwired: 7 in, 2 out]
          }
        }
      }
      frame "Reset Manual Count" {
        w260 = u32 0 ("Rejects")
        n111 = local write "Rejects 2"(w260) -> ()
        n112 = local write "Output Count"(w260) -> ()
      }
      frame "Error" {
        # "Error - Display an error dialog. This message is sent by the \"Error Handler\" VIs at the end of other loops in this application."
        n113 = Variant To Data(error in=w271, type=errorcluster {"status"=FALSE, "code"=0, "source"=""} ("error constant"), Variant=w269) -> (data=w267:errorcluster, error out=w266:errorcluster)
        n114 = call <vilib>:"Simple Error Handler.vi"("error in (no error)"=w267) -> ()  [unwired: 4 in, 5 out]
        n115 = Merge Errors(w266) -> (w265:errorcluster)
      }
      frame "Confirm Quit" {
        # "Confirm Quit - Message that can confirm whether or not the user wants to exit the application."
        n116 = call-poly "Enqueue Message.vi"("Priority Message? (F)"=TRUE, "error in (no error)"=w279, "Message"="Exit", "Message Queue"=w275) -> ("error out"=w276:errorcluster)  [unwired: 6 in, 1 out]
        n117 = Merge Errors(w276) -> (w277:errorcluster)
      }
      frame "Exit" {
        # "Stop the VI"
        # "Release the message queue reference"
        # "Exit - Exit the application."
        n118 = Variant To Data(type=errorcluster {"status"=FALSE, "code"=0, "source"=""} ("error constant"), Variant=w284) -> (data=w285:errorcluster)  [unwired: 1 in, 1 out]
        n119 = call <vilib>:"Simple Error Handler.vi"("error in (no error)"=w285) -> ()  [unwired: 4 in, 5 out]
        n120 = Send Notification(notification=TRUE, notifier=w283) -> (error out=w281:errorcluster)  [unwired: 1 in, 1 out]
        n121 = call "Fire User Event - Stop.vi"("User Event - Stop"=w289) -> ("error out"=w288:errorcluster)  [unwired: 10 in]
        n122 = Release Queue(queue=w294, error in (no error)=w287) -> (error out=w291:errorcluster)  [unwired: 1 in, 2 out]
        n123 = Merge Errors(w281, w288, w291) -> (w290:errorcluster)
      }
      frame Default {
        # "'Default' case only runs if there is a message that isn't defined in any of the other cases.  Output a programming error."
        n124 = xnode "Error Ring"("parameter 0"=w296) -> ("error out"=w297:errorcluster)
      }
    }
    n125 = call "Error Handler - Message Handling Loop.vi"("error in (no error)"=w48, "Message Queue"=w50) -> ("dup error in"=w49:errorcluster)  [unwired: 8 in, 1 out]
  }
  n126 = while {
    tunnel: w28 -> [w313]
    shift-right: [w311] -> w35
    shift-left: w32 -> [w312]
    tunnel: [w307] -> w33
    stop <- w309 stop-if-true
    # "Event Handling Loop"
    n127 = event shown="[13] \"Save Para\": Value Change" {
      selector: w312 -> [_ _ _ _ _ _ _ _ _ _ _ _ _ _ _ _ _ _]
      dyn-events: [_ _ _ _ _ _ _ _ _ _ _ _ _ _ _ _ _ _] -> w311
      timeout: 500 -> [_ _ _ _ _ _ _ _ _ _ _ _ _ _ _ _ _ _]
      tunnel: [_ _ _ _ _ _ _ _ _ _ _ _ _ _ _ _ _ TRUE ("Discard?")] -> w309
      tunnel: w313 -> [w318 w322 w327 w331 w335 w339 w343 w348 w353 w358 w362 w367 w369 w390 w400 w409 w418 w420]
      tunnel: [w317 _ w326 w330 w334 w338 w342 w347 w352 w359 _ w365 w370 w391 _ _ _ _] -> w310
      tunnel: [w316 w322 w325 w329 w333 w337 w341 w346 w351 w358 w362 w366 w369 w390 w400 w409 w418 w420] -> w308
      event Panel Close? {
        n128 = event-data() -> ()  [unwired: 1 in, 1 out]
        n129 = call-poly "Enqueue Message.vi"("Priority Message? (F)"=TRUE, "Message"="Confirm Quit", "Message Queue"=w318) -> ("error out"=w317:errorcluster, "dup Message Queue"=w316:refnum<queue>)  [unwired: 7 in]
        n130 = event-data("Discard?"=TRUE) -> ()  [unwired: 1 in, 1 out]
      }
      event Timeout {
        n131 = event-data() -> ()  [unwired: 1 in, 1 out]
        n132 = Format Date/Time String(time format string (%c)="%d %b %Y | %I:%M:%S %p") -> (date/time string=→"Date-Time":string)  [unwired: 2 in]
      }
      event "Exit": Value Change {
        n133 = event-data() -> ()  [unwired: 1 in, 1 out]
        n134 = call-poly "Enqueue Message.vi"("Priority Message? (F)"=TRUE, "Message"="Exit", "Message Queue"=w327) -> ("error out"=w326:errorcluster, "dup Message Queue"=w325:refnum<queue>)  [unwired: 7 in]
      }
      event "Home Para", "Home Manual": Value Change {
        n135 = event-data() -> ()  [unwired: 1 in, 1 out]
        n136 = call-poly "Enqueue Message.vi"("Message"="Initialize", "Message Queue"=w331) -> ("error out"=w330:errorcluster, "dup Message Queue"=w329:refnum<queue>)  [unwired: 8 in]
      }
      event "Back Stats", "Back IO": Value Change {
        n137 = event-data() -> ()  [unwired: 1 in, 1 out]
        n138 = call-poly "Enqueue Message.vi"("Message"="Autocycle Back", "Message Queue"=w335) -> ("error out"=w334:errorcluster, "dup Message Queue"=w333:refnum<queue>)  [unwired: 8 in]
      }
      event "Stats": Value Change {
        n139 = event-data() -> ()  [unwired: 1 in, 1 out]
        n140 = call-poly "Enqueue Message.vi"("Message"="Autocycle Stats", "Message Queue"=w339) -> ("error out"=w338:errorcluster, "dup Message Queue"=w337:refnum<queue>)  [unwired: 8 in]
      }
      event "All IO": Value Change {
        n141 = event-data() -> ()  [unwired: 1 in, 1 out]
        n142 = call-poly "Enqueue Message.vi"("Message"="Autocycle IO", "Message Queue"=w343) -> ("error out"=w342:errorcluster, "dup Message Queue"=w341:refnum<queue>)  [unwired: 8 in]
      }
      event "Home AC": Value Change {
        n143 = event-data() -> ()  [unwired: 1 in, 1 out]
        n144 = call-poly "Enqueue Message.vi"("Message"="Initialize", "Message Queue"=w348) -> ("error out"=w347:errorcluster, "dup Message Queue"=w346:refnum<queue>)  [unwired: 8 in]
        n145 = call "Write NS (HMI).vi"("Message"="Exit Autocycle") -> ()  [unwired: 10 in, 1 out]
      }
      event "Maintenance", "Parameters", "Manual": Value Change {
        n146 = event-data() -> ("CtlRef"=w350:refnum<vi>)  [unwired: 1 in]
        n147 = property class="Bool"(reference=w350) -> ("Label.Text"=w349:string)  [unwired: 1 in, 2 out]
        n148 = call-poly "Enqueue Message.vi"("Message"=w349, "Message Queue"=w353) -> ("error out"=w352:errorcluster, "dup Message Queue"=w351:refnum<queue>)  [unwired: 8 in]
      }
      event "Enable Insertion?", "Enable Cutting?", "Enable TF?", "Enable PF?", "Enable Index?", "Enable Measure?", "Enable Reject?", "Enable Agitate?", "Enable BF?": Value Change {
        n149 = event-data() -> ("CtlRef"=w360:refnum<vi>, "NewVal"=w354:bool)  [unwired: 1 in, 1 out]
        n150 = property class="Bool (strict)"(reference=w360) -> ("Label.Text"=w357:string)  [unwired: 1 in, 2 out]
        n151 = Concatenate Strings("GV:" ("string"), w357) -> (w355:string)
        n152 = call "Write NS (HMI).vi"("Message Data"=w354, "Message"=w355) -> ("error out"=w359:errorcluster)  [unwired: 9 in]
      }
      event "Reset MCount": Value Change {
        n153 = event-data() -> ()  [unwired: 1 in, 6 out]
        n154 = call-poly "Enqueue Message.vi"("Message"="Reset Manual Count", "Message Queue"=w362) -> ()  [unwired: 8 in, 2 out]
      }
      event "Run Manual": Value Change {
        n155 = event-data() -> ("CtlRef"=w364:refnum<vi>)  [unwired: 1 in, 2 out]
        n156 = property class="Bool"(reference=w364) -> ("Label.Text"=w363:string)  [unwired: 1 in, 2 out]
        n157 = call-poly "Enqueue Message.vi"("Message"=w363, "Message Queue"=w367) -> ("error out"=w365:errorcluster, "dup Message Queue"=w366:refnum<queue>)  [unwired: 8 in]
      }
      event "Toggle Motor": Value Change {
        n158 = event-data() -> ()  [unwired: 1 in, 3 out]
        n159 = call "Write NS (HMI).vi"("Message"="Toggle Motor") -> ("error out"=w370:errorcluster)  [unwired: 10 in]
      }
      event "Save Para": Value Change {
        n160 = event-data() -> ()  [unwired: 1 in, 3 out]
        n161 = Cluster To Array(cluster="Agitator Para") -> (array=w385:u32[])
        n162 = Cluster To Array(cluster="Tube Feeder Para") -> (array=w383:u32[])
        n163 = Cluster To Array(cluster="Insertion Para") -> (array=w381:u32[])
        n164 = Cluster To Array(cluster="Cutting Para") -> (array=w379:u32[])
        n165 = Cluster To Array(cluster="PF Para") -> (array=w377:u32[])
        n166 = Cluster To Array(cluster="Meas. Para") -> (array=w375:dbl[])
        n167 = Cluster To Array(cluster="Reject Para") -> (array=w373:u32[])
        n168 = Cluster To Array(cluster="BF Para") -> (array=w371:u32[])
        n169 = Bundle By Name(cluster=T7 {"Agitator Delays"=[1000], "TF Delays"=[1000], "Insertion Delays"=[1000], "Cutting Delays"=[1000], "PF Delays"=[1000], "Measur. Delays"=[1000.0], "Reject Delays"=[1000], "BF Delays"=[1000]} ("Auto Para"), "Agitator Delays"=w385, "TF Delays"=w383, "Insertion Delays"=w381, "Cutting Delays"=w379, "PF Delays"=w377, "Measur. Delays"=w375, "Reject Delays"=w373, "BF Delays"=w371) -> (w387:T7)
        n170 = call "Write NS (HMI).vi"("Message Data"=w387, "Message"="Save Para") -> ("error out"=w391:errorcluster)  [unwired: 9 in]
      }
      event "Insertion Para.Delay 1", "Insertion Para.Delay 2", "Agitator Para.Delay", "Agitator Para.Timeout", "Cutting Para.Delay", "Cutting Para.Delay 2", "Cutting Para.Delay 3", "Tube Feeder Para.Delay", "Tube Feeder Para.Delay 2", "Tube Feeder Para.Max Attempts", "PF Para.Delay", "PF Para.Timeout", "Reject Para.Delay", "BF Para.Delay 1", "BF Para.Delay 2": Mouse Up {
        n171 = event-data() -> ("CtlRef"=w392:refnum<vi>)  [unwired: 1 in, 4 out]
        n172 = property class="DigNum (strict)"(reference=w392) -> (reference out=w395:refnum<vi>, "Value"=w396:u32)  [unwired: 1 in, 1 out]
        n173 = Number To Fractional String(number=w396, precision (6)=0.0 ("width (-)")) -> (F-format string=w394:string)  [unwired: 2 in]
        n174 = call "HMI Pop Up Num KP v1.1.vi"("String In"=w394) -> ("String Out"=w393:string)  [unwired: 9 in, 1 out]
        n175 = Fract/Exp String To Number(string=w393, default (0 dbl)=0.0 ("default (0 I32)")) -> (number=w398:dbl)  [unwired: 2 in, 1 out]
        n176 = property class="DigNum (strict)"(reference=w395, "Value"=w398) -> ()  [unwired: 1 in, 2 out]
      }
      event "Meas. Para.Delay": Mouse Up {
        n177 = event-data() -> ("CtlRef"=w401:refnum<vi>)  [unwired: 1 in, 4 out]
        n178 = property class="DigNum (strict)"(reference=w401) -> (reference out=w404:refnum<vi>, "Value"=w405:dbl)  [unwired: 1 in, 1 out]
        n179 = Number To Fractional String(number=w405, precision (6)=0.0 ("width (-)")) -> (F-format string=w403:string)  [unwired: 2 in]
        n180 = call "HMI Pop Up Num KP v1.1.vi"("String In"=w403) -> ("String Out"=w402:string)  [unwired: 9 in, 1 out]
        n181 = Fract/Exp String To Number(string=w402, default (0 dbl)=0.0 ("default (0 I32)")) -> (number=w407:dbl)  [unwired: 2 in, 1 out]
        n182 = property class="DigNum (strict)"(reference=w404, "Value"=w407) -> ()  [unwired: 1 in, 2 out]
      }
      event "Meas. Para.Mean Length", "Meas. Para.Tolerance": Mouse Up {
        n183 = event-data() -> ("CtlRef"=w410:refnum<vi>)  [unwired: 1 in, 4 out]
        n184 = property class="DigNum (strict)"(reference=w410) -> (reference out=w413:refnum<vi>, "Value"=w414:dbl)  [unwired: 1 in, 1 out]
        n185 = Number To Fractional String(number=w414, precision (6)=1.0 ("width (-)")) -> (F-format string=w412:string)  [unwired: 2 in]
        n186 = call "HMI Pop Up Num KP v1.1.vi"("String In"=w412) -> ("String Out"=w411:string)  [unwired: 9 in, 1 out]
        n187 = Fract/Exp String To Number(string=w411, default (0 dbl)=0.0 ("default (0 I32)")) -> (number=w416:dbl)  [unwired: 2 in, 1 out]
        n188 = property class="DigNum (strict)"(reference=w413, "Value"=w416) -> ()  [unwired: 1 in, 2 out]
      }
      event User Event {
        # "The Message Handling Loop processed an \"Exit\" message, which fired this event to stop the Event Handling Loop."
        n189 = event-data() -> ()  [unwired: 1 in, 1 out]
      }
    }
    n190 = call "Error Handler - Event Handling Loop.vi"("error in (no error)"=w310, "Message Queue"=w308) -> ("dup error in"=w307:errorcluster)  [unwired: 8 in, 1 out]
  }
  n191 = call "HMI-cRIO Connection Manager.vi"("error in"=w29, "notifier in"=w21, "Queue in"=w28) -> ("error out"=w22:errorcluster, "Notifier out"=w23:refnum<notifier>)  [unwired: 7 in]
  n192 = Unregister For Events(event registration refnum=w35, error in=w33) -> (error out=w36:errorcluster)
  n193 = Merge Errors(w36, w38, w22) -> (w37:errorcluster)
  n194 = call "Destroy User Event - Stop.vi"("error in (no error)"=w37, "User Event - Stop"=w31) -> ("error out"=w25:errorcluster)  [unwired: 9 in]
  n195 = Release Notifier(notifier=w23, error in (no error)=w25) -> (error out=w24:errorcluster)  [unwired: 1 in, 2 out]
  n196 = disable-structure shown="RUN_TIME_ENGINE==True" {
    disable-tunnel: w24 -> [_ _]
    frame condition #0 (active) {
    }
    frame condition #1 {
      # "Call Quit LabVIEW if running as a built application."
      n197 = Quit LabVIEW() -> ()  [unwired: 1 in]
    }
  }
